vi "9605 Field not supported by ObjectType--error.vi"(7 "Clear this error?":bool, 8 "error in":errorcluster, 10 "Field Name":string, 11 "Object Type Base":refnum<class "Object Type Base.lvclass">) -> (0 "error out":errorcluster, 2 "Error Code":i32)   [LabVIEW 2024, in "Electronic Datasheet.lvlib"]
uses:
  Electronic Datasheet.lvlib
  Object Type/Object Type Base.lvclass
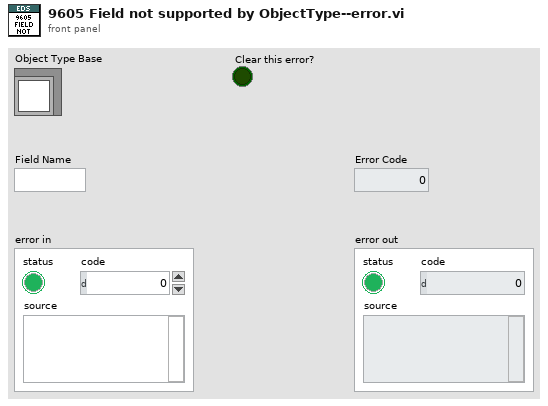
[diagram p1: front panel]
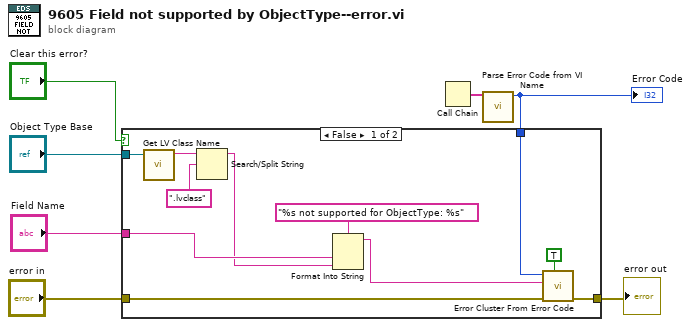
[diagram p0: block diagram]
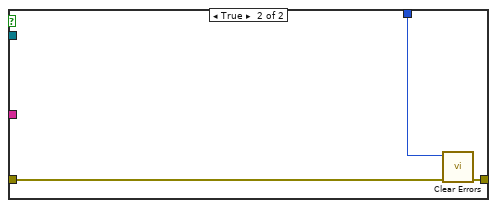
[diagram p2: hidden frame]
diagram:
  n1 = Call Chain() -> (call chain=w2:string[])
  n2 = call "Parse Error Code from VI Name.vi"("Call Chain"=w2) -> ("Error Code"=w1:i32)  [unwired: 10 in]
  "Error Code" <- w1
  n3 = case shown="False" "Clear this error?" {
    tunnel: [w18 w21] -> w7
    tunnel: "Field Name" -> [w16 _]
    tunnel: "Object Type Base" -> [w12 _]
    tunnel: "error in" -> [w10 w20]
    tunnel: w1 -> [w8 w19]
    frame False {
      n4 = call <vilib>:"Get LV Class Name.vi"("object"=w12) -> ("class name"=w14:string)  [unwired: 9 in, 1 out]
      n5 = Search/Split String(string=w14, search string/char (-)=".lvclass") -> (substring before match=w11:string)  [unwired: 1 in, 2 out]
      n6 = Format Into String(format string="%s not supported for ObjectType: %s", w16, w11) -> (resulting string=w9:string)  [unwired: 2 in, 1 out]
      n7 = call <vilib>:"Error Cluster From Error Code.vi"("show call chain? (False)"=TRUE, "error in (no error)"=w10, "error message (\"\")"=w9, "error code (0)"=w8) -> ("error out"=w18:errorcluster)  [unwired: 5 in]
    }
    frame True {
      n8 = call <vilib>:"Clear Errors.vi"("error in (no error)"=w20, "specific error code to clear (0: all)"=w19) -> ("error out"=w21:errorcluster)  [unwired: 4 in, 1 out]
    }
  }
  "error out" <- w7
